vi "Save_Windows_Bounds.vi"(5 "Re-entrant user message window? (F)":bool, 6 "FP.State":T1(ring)=enum."Standard", 7 "Window Name (i.e. Key)":string="Manual Control Menu", 8 "error in":errorcluster, 9 "Front Panel Window:Open":bool, 11 "Window VI's Ref":refnum<vi>) -> (0 "Error out (pass-through)":errorcluster)   [LabVIEW 2020]
uses:
  Typedefs/Window position FG states.ctl
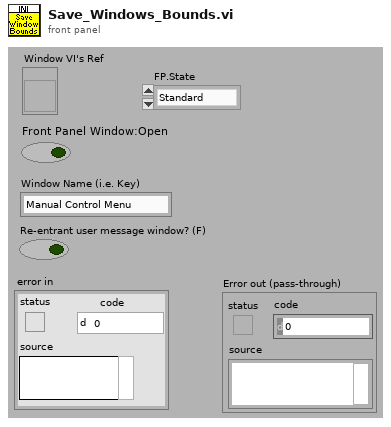
[diagram p1: front panel]
types:
  T1 = enum32{"Invalid", "Standard", "Closed", "Hidden", "Minimized", "Maximized"}
  T2 = typedef "Window position FG states.ctl" = enum16{"Manage", "Query", "Write"}
  T3 = typedef "LVRectTypeDef.ctl" = cluster{"Left":i16, "Top":i16, "Right":i16, "Bottom":i16}
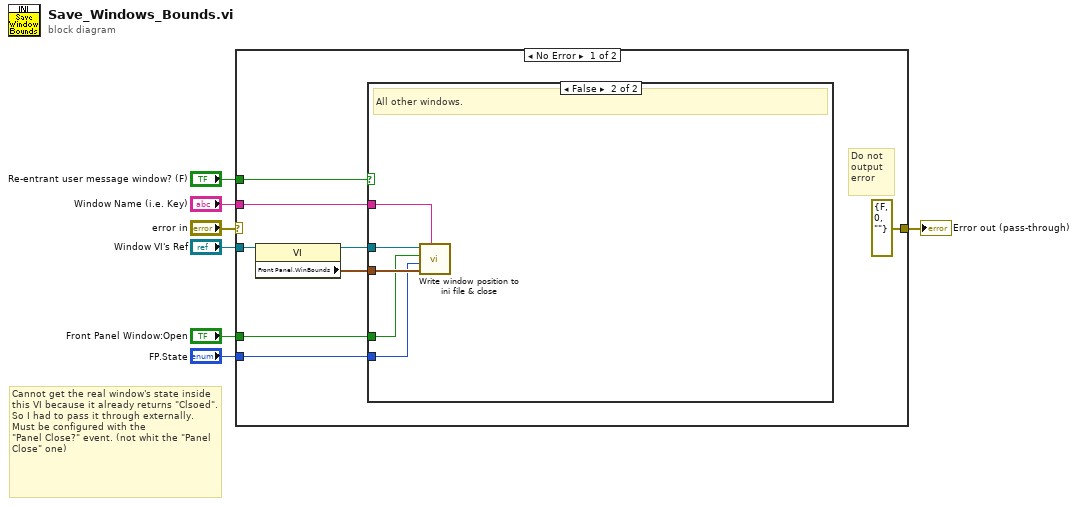
[diagram p0: block diagram]
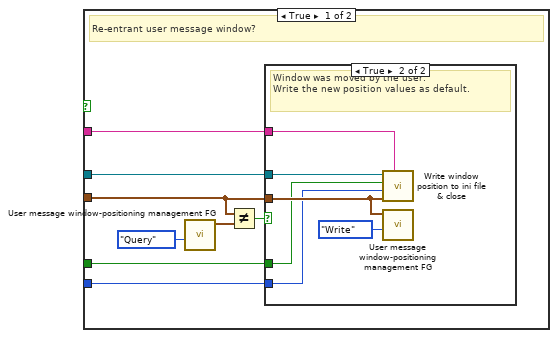
[diagram p2: hidden frame]
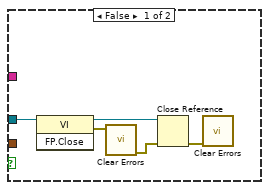
[diagram p3: hidden frame]
diagram:
  # "Cannot get the real window's state inside this VI because it already returns \"Clsoed\". So I had to pass it through externally.\nMust be configured with the \n\"Panel Close?\" event. (not whit the \"Panel Close\" one)"
  n1 = case shown="No Error" "error in" {
    selector: "error in" -> [_ w40]
    tunnel: "Window VI's Ref" -> [w15 _]
    tunnel: "Front Panel Window:Open" -> [w12 _]
    tunnel: [errorcluster {"status"=FALSE, "code"=0, "source"=""} ("error IO") w40] -> w4
    tunnel: "Window Name (i.e. Key)" -> [w13 _]
    tunnel: "Re-entrant user message window? (F)" -> [w11 _]
    tunnel: "FP.State" -> [w8 _]
    frame No Error {
      # "Do not output error"
      n2 = property class="VI"(reference=w15) -> (reference out=w10:refnum<vi>, "Front Panel.WinBounds"=w9:T3)  [unwired: 1 in, 1 out]
      n3 = case shown="False" w11 {
        tunnel: w13 -> [w20 w38]
        tunnel: w12 -> [w19 w36]
        tunnel: w10 -> [w21 w39]
        tunnel: w9 -> [w22 w37]
        tunnel: w8 -> [w16 w35]
        frame True {
          # "Re-entrant user message window?"
          n4 = call "User message window-positioning management FG.vi"("Function (\"Manage\")"=Window_position_FG_states."Query" ("Function (\"Manage\")")) -> ("New window position to set"=w23:T3)  [unwired: 9 in, 1 out]
          n5 = Not Equal?(x=w22, y=w23) -> (x != y?=w18:bool)
          n6 = case shown="True" w18 {
            tunnel: w22 -> [_ w32]
            tunnel: w21 -> [w26 w34]
            tunnel: w20 -> [_ w33]
            tunnel: w19 -> [_ w30]
            tunnel: w16 -> [_ w29]
            frame False {
              n7 = invoke class="VI" method="FP.Close"(reference=w26) -> (reference out=w24:refnum<vi>, error out=w25:errorcluster)  [unwired: 2 in, 1 out]
              n8 = call <vilib>:"Clear Errors.vi"("error in (no error)"=w25) -> ("error out"=w28:errorcluster)  [unwired: 5 in, 1 out]
              n9 = Close Reference(reference=w24, error in (no error)=w28) -> (error out=w27:errorcluster)
              n10 = call <vilib>:"Clear Errors.vi"("error in (no error)"=w27) -> ()  [unwired: 5 in, 2 out]
            }
            frame True {
              # "Window was moved by the user.\nWrite the new position values as default."
              n11 = call "Write window position to ini file & close.vi"("Window Name"=w33, "Front Panel.WinBounds"=w32, "FP.State"=w29, "Disable closing"=w30, "VI in"=w34) -> ()  [unwired: 7 in]
              n12 = call "User message window-positioning management FG.vi"("Function (\"Manage\")"=Window_position_FG_states."Write" ("Function (\"Manage\")"), "Default Window position (in)"=w32) -> ()  [unwired: 8 in, 2 out]
            }
          }
        }
        frame False {
          # "All other windows."
          n13 = call "Write window position to ini file & close.vi"("Window Name"=w38, "Front Panel.WinBounds"=w37, "FP.State"=w35, "Disable closing"=w36, "VI in"=w39) -> ()  [unwired: 7 in]
        }
      }
    }
    frame Error {
    }
  }
  "Error out (pass-through)" <- w4
